vi "KernelCenterer.vi"(8 "error in (no error)":errorcluster caption="entrée d'erreur (pas d'erreur)") -> (0 "error out":errorcluster, 3 "KernelCenterer.lvclass":refnum<class "KernelCenterer.lvclass">)   [LabVIEW 2020]
doc: "Center a kernel matrix\n\nLet K(x, z) be a kernel defined by phi(x)^T phi(z), where phi is a function mapping x to a Hilbert space. KernelCenterer centers (i.e., normalize to have zero mean) the data without explicitly computing phi(x). It is equivalent to centering phi(x) with sklearn.preprocessing.StandardScaler(with_std=False).\n\n\nMethods : \n\n- Fit : Fit KernelCenterer\n\nParameters : K : numpy array of shape [n_samples, n_samples]\n Kernel matrix.\n\n- Fit Transform : Fit to data, then transform it. Fits transformer to X and y with optional parameters fit_params and returns a transformed version of X.\n\nParameters : X : {array-like, sparse matrix, dataframe} of shape (n_samples, n_features)\n y : ndarray of shape (n_samples,), default=None\n Target values.\n\nReturns : X_new : ndarray array of shape (n_samples, n_features_new)\n Transformed array.\n\n\n- Transform : Center kernel matrix.\n\nParameters : K : numpy array of shape [n_samples1, n_samples2]\n Kernel matrix.\n\nReturns : K_new : numpy array of shape [n_samples1, n_samples2]"
uses:
  KernelCenterer.lvclass
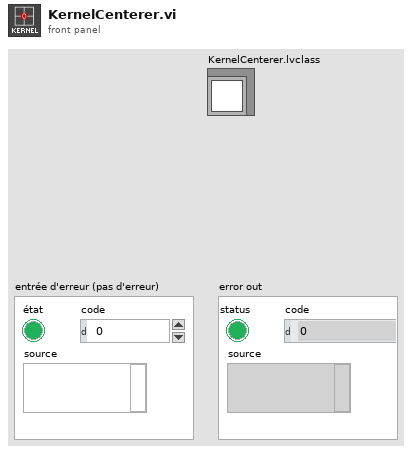
[diagram p1: front panel]
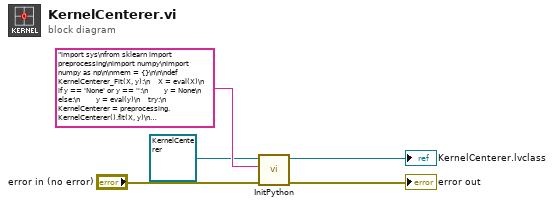
[diagram p0: block diagram]
diagram:
  n1 = call-dynamic "InitPython.vi"("error in (no error)"="error in (no error)", "Python Instruction"="import sys\nfrom sklearn import preprocessing\nimport numpy\nimport numpy as np\n\nmem = {}\n\n\ndef KernelCenterer_Fit(X, y):\n    X = eval(X)\n    if y == 'None' or y == '':\n        y = None\n    else:\n        y = eval(y)\n    try:\n        KernelCenterer = preprocessing.KernelCenterer().fit(X, y)\n        mem['FitKernelCenterer'] = KernelCenterer\n        return str('OK')\n    except:\n        erreur = sys.exc_info()\n        typerr = u\"%s\" % (erreur[0])\n        typerr = typerr[typerr.find(\"'\")+1:typerr.rfind(\"'\")]\n        msgerr = u\"%s\" % (erreur[1])\n        message = str('/!\\\\ {0} : {1}'. format(typerr,msgerr))\n        return message \n    \ndef KernelCenterer_FitTransform(X, y):\n    X = eval(X)\n    if y == 'None' or y == '':\n        y = None\n    else:\n        y = eval(y)\n    try:\n        KernelCenterer = preprocessing.KernelCenterer().fit_transform(X, y)\n        dtype = type(KernelCenterer)\n        if dtype == numpy.ndarray:\n            KernelCenterer = KernelCenterer.tolist()\n            return str(KernelCenterer) \n        else:\n            Mat = KernelCenterer.tocoo()\n            return str(list(zip(Mat.row, Mat.col, Mat.data)))\n    except:\n        erreur = sys.exc_info()\n        typerr = u\"%s\" % (erreur[0])\n        typerr = typerr[typerr.find(\"'\")+1:typerr.rfind(\"'\")]\n        msgerr = u\"%s\" % (erreur[1])\n        message = str('/!\\\\ {0} : {1}'. format(typerr,msgerr))\n        return message \n\ndef KernelCenterer_Transform(K, y):\n    K = eval(K)\n    if y == 'None' or y == '':\n        y = None\n    else:\n        y = eval(y)\n    try:\n        KernelCenterer = mem['FitKernelCenterer'].transform(K)\n        dtype = type(KernelCenterer)\n        if dtype == numpy.ndarray:\n            KernelCenterer = KernelCenterer.tolist()\n            return str(KernelCenterer) \n        else:\n            Mat = KernelCenterer.tocoo()\n            return str(list(zip(Mat.row, Mat.col, Mat.data)))\n    except:\n        erreur = sys.exc_info()\n        typerr = u\"%s\" % (erreur[0])\n        typerr = typerr[typerr.find(\"'\")+1:typerr.rfind(\"'\")]\n        msgerr = u\"%s\" % (erreur[1])\n        message = str('/!\\\\ {0} : {1}'. format(typerr,msgerr))\n        return message ", "Scikit-learn en entrée"=refnum<class "KernelCenterer.lvclass"> refnum ("KernelCenterer.lvclass")) -> ("error out"=→"error out":errorcluster, "Scikit-learn en sortie"=→"KernelCenterer.lvclass":refnum<class "KernelCenterer.lvclass">)  [unwired: 7 in]
